vi "niDTS WLAN INSTR RX CLS.vi"(8 "error in (no error)":errorcluster, 11 "niDTS WLAN INSTR RX in":refnum<class "niDTS WLAN INSTR RX.lvclass">) -> (0 "error out":errorcluster, 3 "niDTS WLAN INSTR RX out":refnum<class "niDTS WLAN INSTR RX.lvclass">)   [LabVIEW 2015, in "niDTS WLAN.lvlib" / "niDTS WLAN INSTR RX.lvclass"]
uses:
  niDTS WLAN INSTR RX.lvclass
  RiviInstDriver/niRfsgWlan/Objects/niRfsgWlan.lvclass
  RiviInstDriver/InstDriver/Objects/InstDriver.lvclass
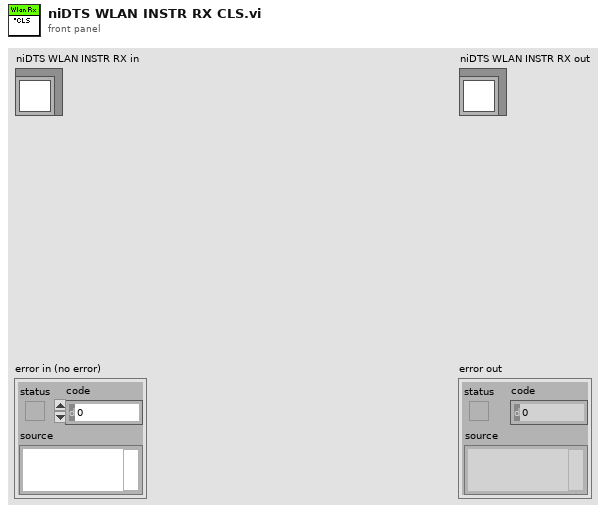
[diagram p1: front panel]
types:
  T1 = typedef "niRfsgWlan.lvclass/niRfsgWlan INC Handle.ctl" = refnum<data-value>
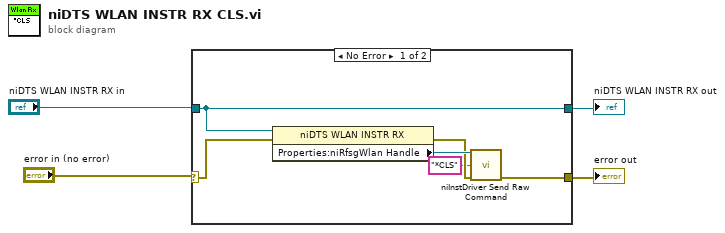
[diagram p0: block diagram]
diagram:
  n1 = case shown="No Error" "error in (no error)" {
    selector: "error in (no error)" -> [w9 w12]
    tunnel: [w5 w12] -> w2
    tunnel: [w10 w11] -> w1
    tunnel: "niDTS WLAN INSTR RX in" -> [w10 w11]
    frame No Error {
      n2 = property class="niDTS WLAN INSTR RX"(reference=w10, error in=w9) -> (error out=w7:errorcluster, "Properties:niRfsgWlan Handle"=w8:T1)  [unwired: 1 out]
      n3 = call "niInstDriver Send Raw Command.vi"("InstDriver Handle in"=w8, "Command"="*CLS", "error in (no error)"=w7) -> ("error out"=w5:errorcluster)  [unwired: 11 in, 1 out]
    }
    frame Error {
    }
  }
  "error out" <- w2
  "niDTS WLAN INSTR RX out" <- w1
